vi "Image_Snap_Dual.vi"(8 "error in":errorcluster, 10 "input cluster":T1={"L16 Linear Actuator"="ASRL6::INSTR", "XE 1000 Pump"="COM10", "Camera1"="cam2", "Camera2"="cam3", "Camera1_IMG"="remote image 0000000015E6FBB4", "Camera2_IMG"="remote image 0000000015E6F134", "Img_Capt"=TRUE, "Actuator"=TRUE, "Pump"=TRUE, "Cam 1"=TRUE, "Cam 2"=TRUE, "Empty_Refill"=FALSE, "Crop"=TRUE, "Light intensity"=50, "Exposure Time"=1000.0, "Sample Name"="Test Sample", "Operator"="MRJ", "Calibration 1"=path "C:/Users/au540322/Desktop/IHS_Project/calibration/Test Calibration/Test Calibration_7/1Test Calibration_7_2019_06_07-23-38-32-452.PNG", "Calibration 2"=path "C:/Users/au540322/Desktop/IHS_Project/calibration/Test Calibration/Test Calibration_7/2Test Calibration_7_2019_06_07-23-38-32-415.PNG", "Framerate"=1, "Timeout Sample"=50, "Collection date"="First test samples", "Sample size threshold"=1, "Empty start"=1, "Command"="MRJ", "Calibration Image 1"=refnum, "Calibration Image 2"=refnum, "Original Image 1"=refnum, "Original Image 2"=refnum, "Processing Image 1"=refnum, "Processing Image 2"=refnum, "Object Image 1"=refnum, "Object Image 2"=refnum, "Cam 1 - save queue"=refnum, "Cam 2 - save queue"=refnum, "Station"="", "Species Name"="", "Other Notes"="", "Aperture"=enum."Item 0", "Image Process Queue Size"=500, "Image Save Queue Size"=500, "Overload threshold"=500, "Max Framerate"=100, "Blue Plane Image"=refnum, "Subtract Image"=refnum, "Binary Image 1"=refnum, "ROI mask allocation"=refnum, "Rectangle 1"={"Left"=0, "Top"=0, "Right"=0, "Bottom"=0, "Rotation"=0.0}, "Rectangle 2"={"Left"=0, "Top"=0, "Right"=0, "Bottom"=0, "Rotation"=0.0}, "Binary Image 2"=refnum, "Detection Region %"=0.0, "Cam 1 queue"=refnum, "Cam 2 queue"=refnum, "Detect image 1"=refnum, "Detect image 2"=refnum, "Detect 1"=path "C:/Users/au540322/Desktop/IHS_Project/images/Debris/Debris_0/Debris_0_2019_06_01-23-32-49-686.PNG", "Detect 2"=path "C:/Users/au540322/Desktop/IHS_Project/images/Debris/Debris_0/Debris_0_2019_06_01-23-32-49-686.PNG", "Max large object threshold"=0, "Open(T)/Close(F)"=FALSE} {"Rectangle 2"."Rotation" format="%.2f"; "Rectangle 2"."Left" scale=0.0..1024.0; "Rectangle 2"."Right" scale=0.0..1024.0; "Rectangle 1"."Rotation" format="%.2f"; "Rectangle 1"."Left" scale=0.0..1024.0; "Rectangle 1"."Right" scale=0.0..1024.0; "Max Framerate" min=1; "Overload threshold" min=1; "Image Save Queue Size" min=1; "Image Process Queue Size" min=1; "Empty start" min=1; "Sample size threshold" min=1; "Framerate" min=1; "Light intensity" scale=0.0..100.0}, 11 "Detect Movement":bool) -> (0 "error out":errorcluster, 1 "Image2":T3, 2 "Image1":T3, 3 "Framerate":i32)   [LabVIEW 2019]
doc: "Gather pictures from both cameras, returns two picture arrays."
uses:
  <vilib>/vision/Image Controls.llb/IMAQ Image.ctl
  controls/Data.ctl
  <vilib>/userdefined/High Color/IMAQdx.ctl
  <vilib>/vision/driver/IMAQdx.llb/IMAQdx Acquisition Mode.ctl
  Camera_ID.ctl
  <vilib>/vision/driver/NI_Vision_Acquisition_Software.lvlib
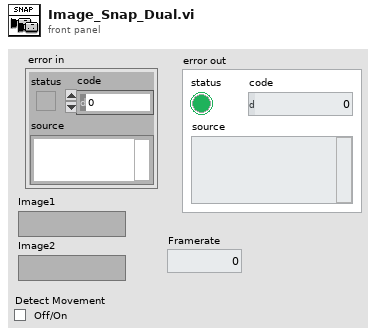
[diagram p1: front panel]
types:
  T1 = typedef "Data.ctl" = cluster{"L16 Linear Actuator":refnum<visa-resource-name>, "XE 1000 Pump":refnum<visa-resource-name>, "Camera1":T2, "Camera2":T2, "Camera1_IMG":T3, "Camera2_IMG":T3, "Img_Capt":bool, "Actuator":bool, "Pump":bool, "Cam 1":bool, "Cam 2":bool, "Empty_Refill":bool, "Crop":bool, "Light intensity":i32, "Exposure Time":dbl, "Sample Name":string, "Operator":string, "Calibration 1":path, "Calibration 2":path, "Framerate":i32, "Timeout Sample":i32, "Collection date":string, "Sample size threshold":i32, "Empty start":u32, "Command":string, "Calibration Image 1":T3, "Calibration Image 2":T3, "Original Image 1":T3, "Original Image 2":T3, "Processing Image 1":T3, "Processing Image 2":T3, "Object Image 1":T3, "Object Image 2":T3, "Cam 1 - save queue":refnum<queue>, "Cam 2 - save queue":refnum<queue>, "Station":string, "Species Name":string, "Other Notes":string, "Aperture":enum32{"Item 0", "Item 1", "Item 2", "Item 3"}, "Image Process Queue Size":i32, "Image Save Queue Size":i32, "Overload threshold":i32, "Max Framerate":i32, "Blue Plane Image":T3, "Subtract Image":T3, "Binary Image 1":T3, "ROI mask allocation":T3, "Rectangle 1":T4, "Rectangle 2":T4, "Binary Image 2":T3, "Detection Region %":dbl, "Cam 1 queue":refnum<queue>, "Cam 2 queue":refnum<queue>, "Detect image 1":T3, "Detect image 2":T3, "Detect 1":path, "Detect 2":path, "Max large object threshold":i32, "Open(T)/Close(F)":bool}
  T2 = typedef "IMAQdx.ctl" = refnum<k21>
  T3 = typedef "IMAQ Image.ctl" = refnum<image>
  T4 = typedef "IMAQ Rectangle" = cluster{"Left":i32, "Top":i32, "Right":i32, "Bottom":i32, "Rotation":dbl}
  T5 = typedef "NI_Vision_Acquisition_Software.lvlib/IMAQdx Acquisition Mode.ctl" = enum32{"One Shot", "Continuous"}
  T6 = typedef "Camera_ID.ctl" = enum16{"Camera 1", "Camera 2"}
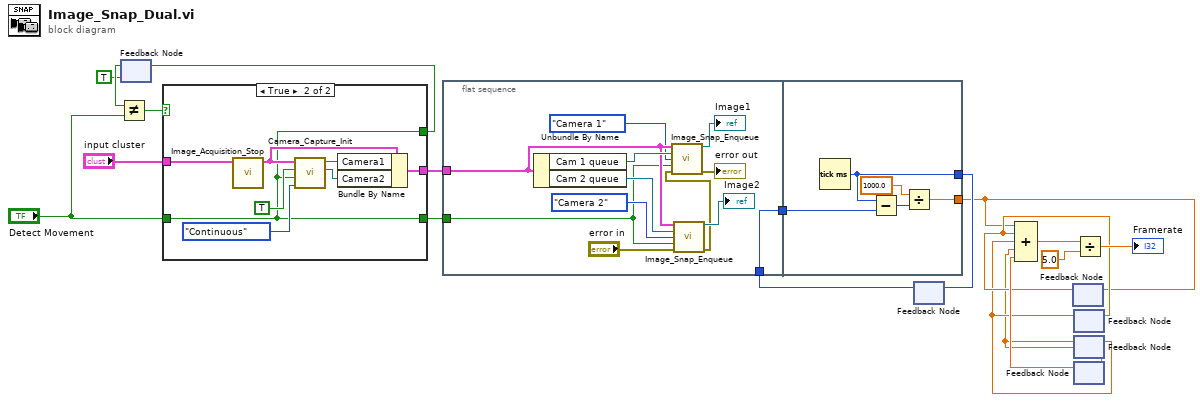
[diagram p0: block diagram]
diagram:
  n1 = feedback #1(TRUE ("Detect Movement")) -> (w5:bool)
  n2 = Not Equal?(x=w5, y="Detect Movement") -> (x != y?=w6:bool)
  n3 = case shown="True" w6 {
    tunnel: "input cluster" -> [w21 w24]
    tunnel: "Detect Movement" -> [w20 w22]
    tunnel: [w20 w22] -> w4
    tunnel: [w21 w23] -> w3
    tunnel: [w20 w22] -> w2
    frame False {
    }
    frame True {
      n4 = call "Image_Acquisition_Stop.vi"("input cluster"=w24) -> ("Output cluster"=w25:T1)  [unwired: 10 in]
      n5 = call "Camera_Capture_Init.vi"("Continuous?"=IMAQdx_Acquisition_Mode."Continuous", "Detect Movement"=w22, "Crop?"=TRUE, "input cluster"=w25) -> ("Camera2"=w26:T2, "Camera1"=w27:T2)  [unwired: 6 in]
      n6 = Bundle By Name(cluster=w25, "Camera1"=w27, "Camera2"=w26) -> (w23:T1)
    }
  }
  n7 = feedback-in #1(w4) -> ()
  n8 = flat-sequence {
    tunnel: [w34] -> w19
    tunnel: w17 -> [w34]
    tunnel: w3 -> [w33]
    tunnel: w2 -> [w30]
    tunnel: w19 -> [w46]
    tunnel: [w45] -> w18
    tunnel: [w42] -> w9
    frame #0 {
      n9 = Unbundle By Name(w33) -> ("Cam 1 queue"=w37:refnum<queue>, "Cam 2 queue"=w36:refnum<queue>)
      n10 = call "Image_Snap_Enqueue.vi"("input cluster"=w33, "queue"=w36, "Camera"=Camera_ID."Camera 2", "Detect Movement"=w30, "error in"="error in") -> ("Image out"=→"Image2":T3, "error out"=w35:errorcluster)  [unwired: 9 in]
      n11 = call "Image_Snap_Enqueue.vi"("input cluster"=w33, "queue"=w37, "Camera"=Camera_ID."Camera 1", "Detect Movement"=w30, "error in"=w35) -> ("Image out"=→"Image1":T3, "error out"=→"error out":errorcluster)  [unwired: 9 in]
    }
    frame #1 {
      n12 = Tick Count (ms)() -> (millisecond timer value=w45:u32)
      n13 = Subtract(x=w45, y=w46) -> (x-y=w44:u32)
      n14 = Divide(x=1000.0, y=w44) -> (x/y=w42:dbl)
    }
  }
  n15 = feedback #2() -> (w17:u32)  [unwired: 1 in]
  n16 = feedback-in #2(w18) -> ()
  n17 = feedback #3() -> (w12:dbl)  [unwired: 1 in]
  n18 = feedback-in #3(w9) -> ()
  n19 = feedback #4() -> (w11:dbl)  [unwired: 1 in]
  n20 = feedback-in #4(w12) -> ()
  n21 = feedback #5() -> (w10:dbl)  [unwired: 1 in]
  n22 = feedback-in #5(w11) -> ()
  n23 = feedback #6() -> (w13:dbl)  [unwired: 1 in]
  n24 = Compound Arithmetic op=ADD(w9, w12, w11, w10, w13) -> (w16:dbl)
  n25 = feedback-in #6(w10) -> ()
  n26 = Divide(x=w16, y=5.0) -> (x/y=→"Framerate":dbl)
